vi "PLC OPC Prototype.vi"() -> ()   [LabVIEW 2013]
uses:
  Sub VIs/OPC Engine/Controls/ALTS-2015 OPC Write Registers.ctl
  Sub VIs/OPC Engine/Controls/ALTS-2015 OPC Read Registers.ctl
  Sub VIs/OPC Engine/Controls/ALTS-2015 OPC Read Global Options.ctl
  Sub VIs/OPC Engine/Controls/ALTS-2015 OPC Write Global Options.ctl
  Sub VIs/OPC Engine/Globals/ALTS-2015 OPC Engine Globals.vi
panel:
  in  "Flage Size":string
  in  "OPC Write Single":T1=enum."Serial_Flange_Size"
  in  "OPC Read Register Array":T2[](array[typedef])=[enum."Robot_Available", enum."Start_Test", enum."Stop_Test", enum."Scan_Trigger"]
  out "OPC Read Register Array Value":variant[](array[variant])=[variant(i32 0), variant(i32 0), variant(i32 0), variant(i32 0)]
  out "Read Values":i32[](array[numeric])
  in  "OPC Write Register Array":T1[](array[typedef])=[enum."Task_Available_for_Robot", enum."New_Serial", enum."Serial_Adapter_Size", enum."Serial_Displacement_Size", enum."Serial_Flange_Size", enum."Test_Result", enum."Test_Result", enum."Station_Number", enum."Rerun", enum."Invalid_SNo"]
  in  "Write Values":i32[](array[numeric])=[1, 0, 1, 0, 1, 0, 1, 0, 1, 0]
  in  "Read Registers":string[](array[string])=["[Master_PLC]DACS_TS1_Air_Leak_Test_Not_Passed", "[Master_PLC]DACS_TS1_Repair_Code_Missing", "[Master_PLC]DACS_TS1_Estop_Alarm_Light"]
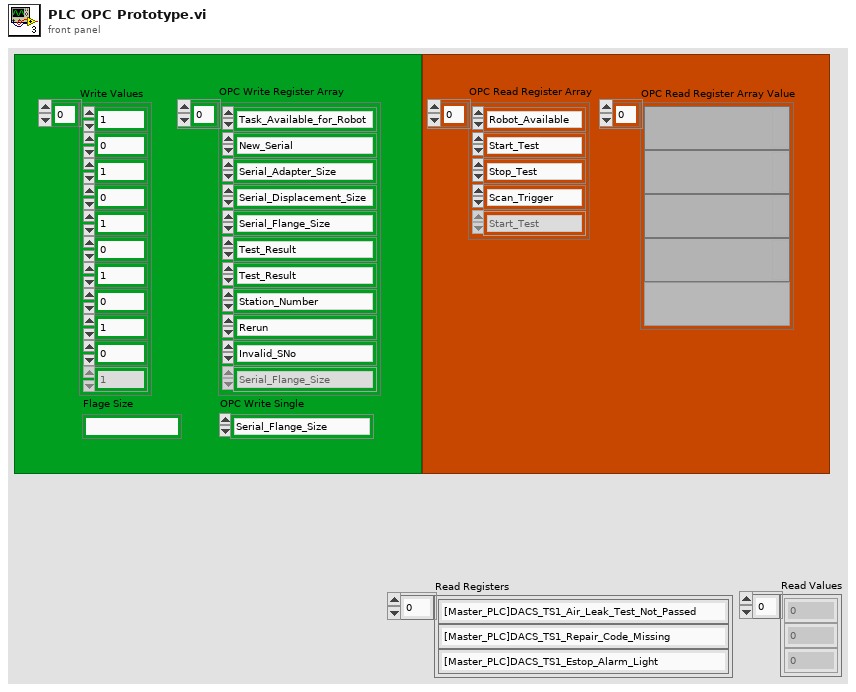
[diagram p1: front panel]
types:
  T1 = typedef "ALTS-2015 OPC Write Registers.ctl" = enum16{"Task_Available_for_Robot", "New_Serial", "Serial_Adapter_Size", "Serial_Displacement_Size", "Serial_Flange_Size", "Test_Result", "Station_Number", "Rerun", "Invalid_SNo", "PC_ACK_Read_Tags"}
  T2 = typedef "ALTS-2015 OPC Read Registers.ctl" = enum16{"Robot_Available", "Start_Test", "Stop_Test", "Scan_Trigger", "Station_No_Start_Stop_Test"}
  T3 = enum16{"Read", "Write", "ReadWrite", "BufferedRead", "BufferedReadWrite"}
  T4 = typedef "ALTS-2015 OPC Write Global Options.ctl" = enum16{"Init", "Write Value", "Write Array", "Read Value", "Read Array", "Read All"}
  T5 = typedef "ALTS-2015 OPC Read Global Options.ctl" = enum16{"Init", "Write Value", "Write Array", "Read Value", "Read Array", "Read All"}
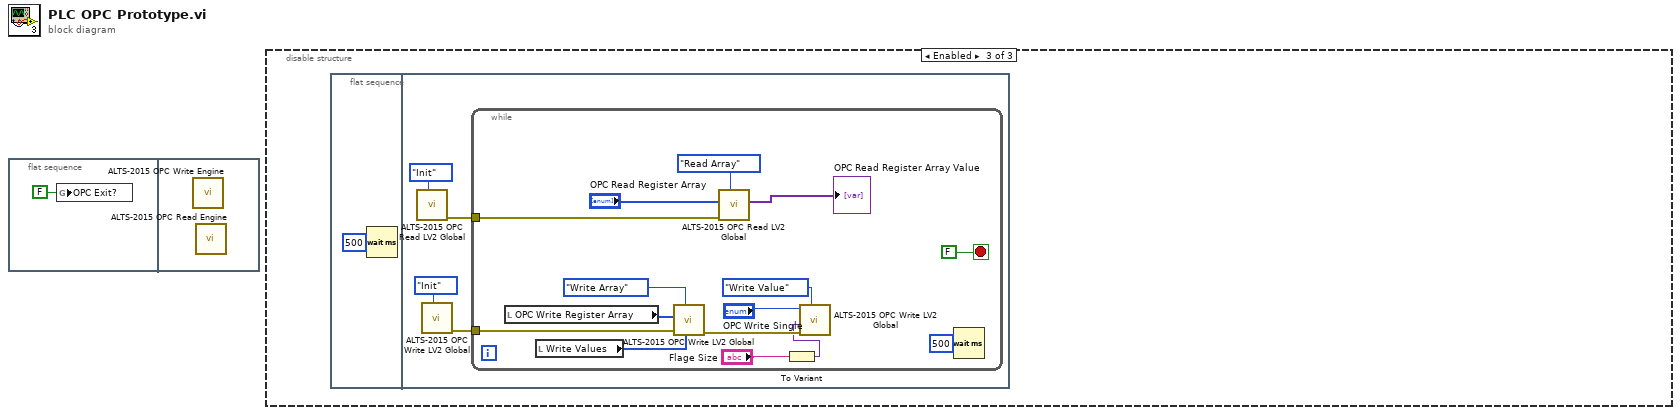
[diagram p0: block diagram]
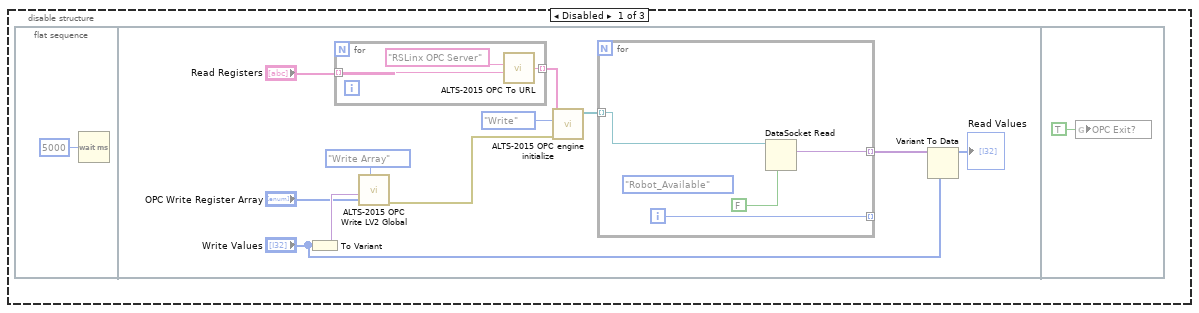
[diagram p2: hidden frame]
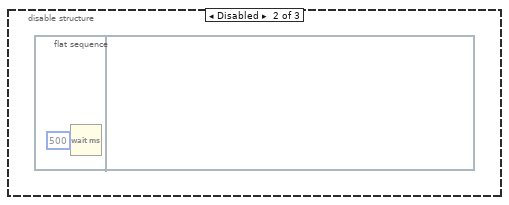
[diagram p3: hidden frame]
diagram:
  n1 = flat-sequence {
    frame #0 {
      n2 = global write "ALTS-2015 OPC Engine Globals.vi" "OPC Exit?"(FALSE ("OPC Exit?")) -> ()
    }
    frame #1 {
      n3 = call "ALTS-2015 OPC Write Engine.vi"() -> ()  [unwired: 11 in, 1 out]
      n4 = call "ALTS-2015 OPC Read Engine.vi"() -> ()  [unwired: 11 in, 1 out]
    }
  }
  n5 = disable-structure shown="Enabled" {
    frame Disabled {
      n6 = flat-sequence {
        frame #0 {
          n7 = Wait (ms)(milliseconds to wait=u32 5000) -> ()  [unwired: 1 out]
        }
        frame #1 {
          n8 = To Variant(anything="Write Values") -> (Variant=w12:variant)
          n9 = for {
            tunnel: "Read Registers" -> [w20] mode=indexing
            tunnel: [w19] -> w11 mode=indexing
            n10 = call "ALTS-2015 OPC To URL.vi"("Item Name"=w20, "Server Name"="RSLinx OPC Server") -> ("URL"=w19:string)  [unwired: 4 in]
          }
          n11 = call "ALTS-2015 OPC Write LV2 Global.vi"("Options"=ALTS-2015_OPC_Write_Global_Options."Write Array", "OPC value"=w12, "OPC Write Register Array"="OPC Write Register Array") -> ("error out"=w3:errorcluster)  [unwired: 6 in, 2 out]
          n12 = call "ALTS-2015 OPC engine initialize.vi"("error in (no error)"=w3, "mode"=T3."Write", "URLs"=w11) -> ("Connection ids"=w8:refnum<k13>[])  [unwired: 7 in, 1 out]
          n13 = for {
            tunnel: [w17] -> w7 mode=indexing
            tunnel: [w15] -> _ mode=indexing
            tunnel: w8 -> [w14] mode=indexing
            i -> [w15]
            (unwired) ALTS-2015_OPC_Read_Registers."Robot_Available" ("Read Register")
            n14 = DataSocket Read(6:FALSE ("wait for updated value (T)"), 11:w14) -> (2:w17:variant)  [unwired: 3 in, 6 out]
          }
          n15 = Variant To Data(type="Write Values", Variant=w7) -> (data=→"Read Values":i32[])  [unwired: 1 in, 1 out]
        }
        frame #2 {
          n16 = global write "ALTS-2015 OPC Engine Globals.vi" "OPC Exit?"(TRUE ("OPC Exit?")) -> ()
        }
      }
    }
    frame Disabled {
      n17 = flat-sequence {
        frame #0 {
          n18 = Wait (ms)(milliseconds to wait=u32 500) -> ()  [unwired: 1 out]
        }
        frame #1 {
        }
      }
    }
    frame Enabled {
      n19 = flat-sequence {
        frame #0 {
          n20 = Wait (ms)(milliseconds to wait=u32 500) -> ()  [unwired: 1 out]
        }
        frame #1 {
          n21 = call "ALTS-2015 OPC Read LV2 Global.vi"("Options"=ALTS-2015_OPC_Read_Global_Options."Init") -> ("error out"=w27:errorcluster)  [unwired: 8 in, 2 out]
          n22 = call "ALTS-2015 OPC Write LV2 Global.vi"("Options"=ALTS-2015_OPC_Write_Global_Options."Init") -> ("error out"=w24:errorcluster)  [unwired: 8 in, 2 out]
          n23 = while {
            tunnel: w27 -> [w42]
            tunnel: w24 -> [w36]
            stop <- FALSE stop-if-true
            n24 = local read "OPC Write Register Array"() -> (w35:T1[])
            n25 = local read "Write Values"() -> (w33:i32[])
            n26 = call "ALTS-2015 OPC Write LV2 Global.vi"("OPC value Array"=w33, "Options"=ALTS-2015_OPC_Write_Global_Options."Write Array", "error in (no error)"=w36, "OPC Write Register Array"=w35) -> ("error out"=w32:errorcluster)  [unwired: 5 in, 2 out]
            n27 = call "ALTS-2015 OPC Read LV2 Global.vi"("Options"=ALTS-2015_OPC_Read_Global_Options."Read Array", "error in (no error)"=w42, "OPC Read Register Array"="OPC Read Register Array") -> ("OPC Read Register Array Value"=→"OPC Read Register Array Value":variant[])  [unwired: 6 in, 2 out]
            n28 = To Variant(anything="Flage Size") -> (Variant=w29:variant)
            n29 = call "ALTS-2015 OPC Write LV2 Global.vi"("Options"=ALTS-2015_OPC_Write_Global_Options."Write Value", "error in (no error)"=w32, "OPC value"=w29, "OPC Write Register"="OPC Write Single") -> ()  [unwired: 5 in, 3 out]
            n30 = Wait (ms)(milliseconds to wait=u32 500) -> ()  [unwired: 1 out]
          }
        }
      }
    }
  }
